vi "Recording.vi"(6 "Measurement Results In":T1 {"Actual Record Length" format="%#_6p Samples"; "Actual Record Duration" format="%#_6p Samples"; "Actual Sample Rate" format="%#_6ps"}, 7 "Recording Settings":T2={"Number of Records"=0, "Plot Names"=[], "Stream To File?"=FALSE, "TDMS Session"=refnum, "Fetch Timeout"=0.0, "Channels Per Record"=1} {"Fetch Timeout" format="%.2f"}, 8 "error in":errorcluster, 9 "Channel List":string, 10 "FGEN Session In":refnum<k15>, 11 "measurement context in":refnum<class "Measure Call Context.lvclass">) -> (0 "error out":errorcluster, 3 "measurement context out":refnum<class "Measure Call Context.lvclass">, 4 "Measurement Results Out":T1 {"Actual Record Length" format="%#_6p Samples"; "Actual Record Duration" format="%#_6ps"; "Actual Sample Rate" format="%#_6pHz"})   [LabVIEW 2025, in "Ni-Scope-Multirecords.lvclass"]
uses:
  Ni-Scope-Multirecords.lvclass
  Recording Settings.ctl
  <vilib>/Plug-In SDKs/Measurements/Measure Call Context/Measure Call Context.lvclass
  Measurement Results.ctl
  Wfm Data.ctl
  <extravilib>/ChannelInstances/Stream-t'Ni-Scope-Multirecords.lvclass-Wfm Data.ctl'/Read.vi
  <extravilib>/ChannelInstances/Stream-t'Ni-Scope-Multirecords.lvclass-Wfm Data.ctl'/Write With Abort.vi
  <extravilib>/ChannelInstances/Stream-t'Ni-Scope-Multirecords.lvclass-Wfm Data.ctl'/Read With Abort.vi
  <extravilib>/ChannelInstances/Stream-t'Ni-Scope-Multirecords.lvclass-Wfm Data.ctl'/Endpoint.vi
  <extravilib>/ChannelInstances/Stream-t'Ni-Scope-Multirecords.lvclass-Wfm Data.ctl'/EndpointRead.vi
  <extravilib>/ChannelInstances/Stream-t'Ni-Scope-Multirecords.lvclass-Wfm Data.ctl'/Instantiate.vi
  <extravilib>/ChannelInstances/Stream-t'Ni-Scope-Multirecords.lvclass-Wfm Data.ctl'/)Channel.vi
  <resource>/ChannelSupport/_ChannelSupport/WaitIfNeeded.vi
  <instrlib>/niScope/Acquire/Fetch/niScope Multi Fetch Cluster.vi
  Ni-Scope-Multirecords.lvclass/Ni-Scope-Multirecords.ctl
  <extravilib>/ChannelInstances/Stream-t'Ni-Scope-Multirecords.lvclass-Wfm Data.ctl'.lvlib
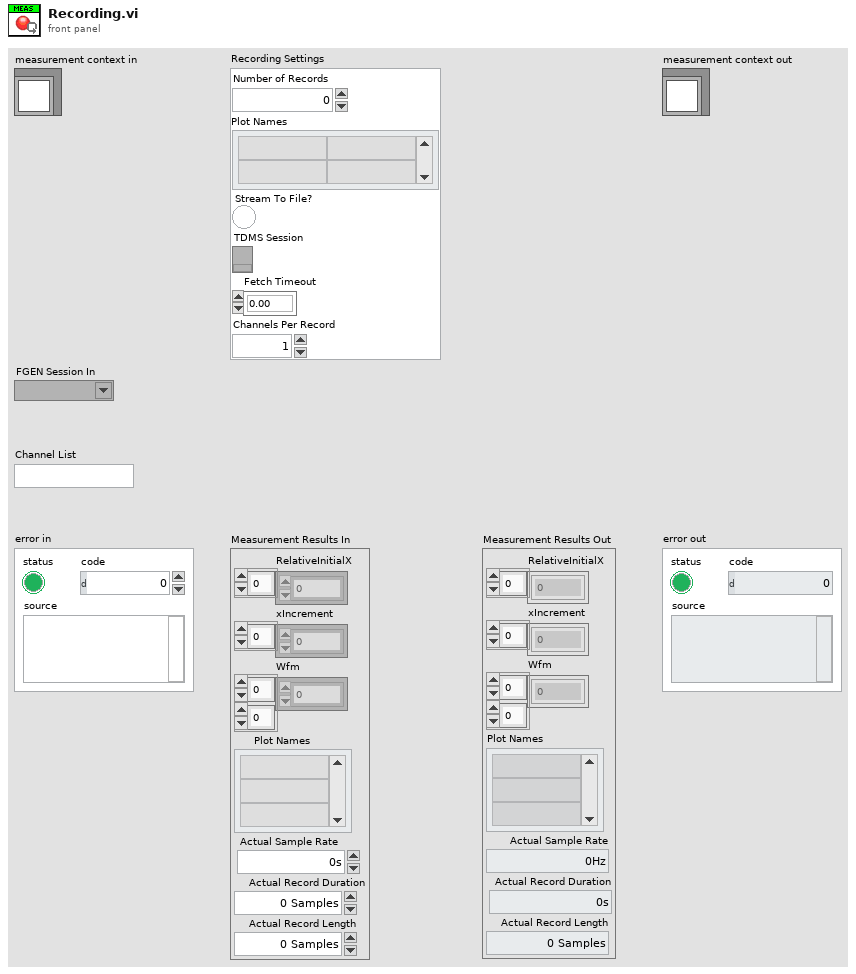
[diagram p1: front panel]
types:
  T1 = typedef "Ni-Scope-Multirecords.lvclass/Measurement Results.ctl" = cluster{"RelativeInitialX":dbl[], "xIncrement":dbl[], "Wfm":dbl[][], "Plot Names":string[], "Actual Sample Rate":dbl, "Actual Record Duration":dbl, "Actual Record Length":dbl}
  T2 = typedef "Ni-Scope-Multirecords.lvclass/Recording Settings.ctl" = cluster{"Number of Records":i32, "Plot Names":string[][], "Stream To File?":bool, "TDMS Session":refnum<k34>, "Fetch Timeout":dbl, "Channels Per Record":i32}
  T3 = typedef "Ni-Scope-Multirecords.lvclass/Wfm Data.ctl" = cluster{"waveform":cluster{"relativeInitialX":dbl, "xIncrement":dbl, "wfm":dbl[]}[]}
  T4 = cluster{"relativeInitialX":dbl, "xIncrement":dbl, "wfm":dbl[]}[]
  T5 = typedef "Stream-t'Ni-Scope-Multirecords.lvclass-Wfm Data.ctl'.lvlib/)Channel.ctl" = refnum<queue>
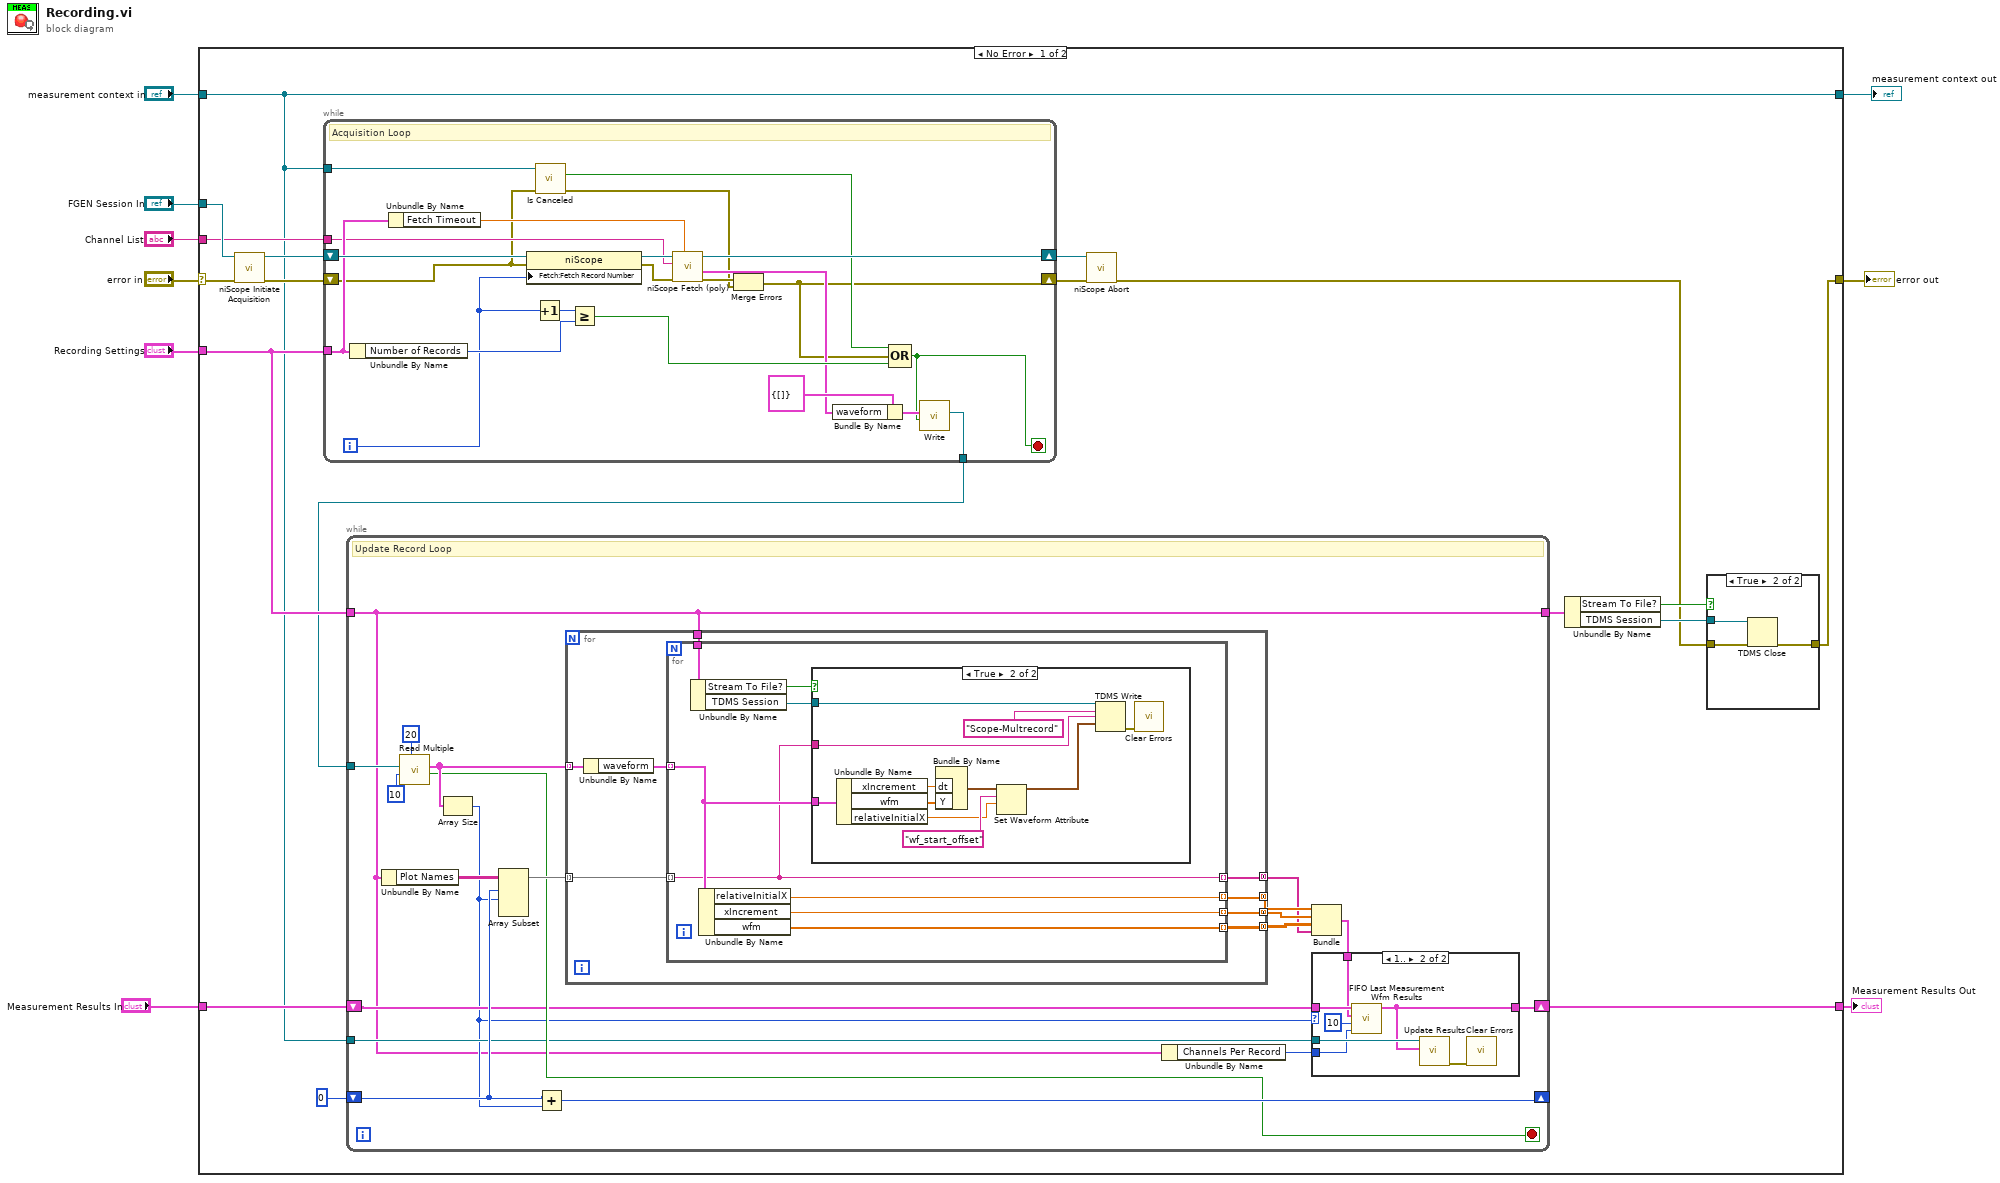
[diagram p0: block diagram]
diagram:
  n1 = case shown="No Error" "error in" {
    selector: "error in" -> [w27 w111]
    tunnel: [w10 w111] -> w8
    tunnel: "Recording Settings" -> [w23 _]
    tunnel: "measurement context in" -> [w17 w110]
    tunnel: "FGEN Session In" -> [w25 _]
    tunnel: [w17 w110] -> w4
    tunnel: "Channel List" -> [w19 _]
    tunnel: "Measurement Results In" -> [w18 w109]
    tunnel: [w16 w109] -> w1
    frame No Error {
      n2 = call <instrlib>:"niScope Initiate Acquisition.vi"("instrument handle"=w25, "error in"=w27) -> ("instrument handle out"=w26:refnum<k15>, "error out"=w24:errorcluster)  [unwired: 12 in]
      n3 = while {
        tunnel: w23 -> [w100]
        shift-right: [w106] -> w15
        shift-left: w26 -> [w108]
        shift-right: [w88] -> w20
        shift-left: w24 -> [w89]
        tunnel: w17 -> [w97]
        tunnel: [w93] -> w22
        tunnel: w19 -> [w91]
        i -> [w103]
        stop <- w92 stop-if-true
        # "Acquisition Loop"
        n4 = Unbundle By Name(w100) -> ("Number of Records"=w105:i32)
        n5 = Unbundle By Name(w100) -> ("Fetch Timeout"=w99:dbl)
        n6 = property class="niScope"(reference=w108, error in=w89, "Fetch:Fetch Record Number"=w103) -> (reference out=w107:refnum<k15>, error out=w101:errorcluster)
        n7 = Increment(x=w103) -> (x+1=w104:i32)
        n8 = call <vilib>:"Is Canceled.vi"("error in"=w89, "measure call context in"=w97) -> ("error out"=w87:errorcluster, "is canceled?"=w90:bool)  [unwired: 7 in, 1 out]
        n9 = Greater Or Equal?(x=w104, y=w105) -> (x >= y?=w102:bool)
        n10 = call-poly <instrlib>:"niScope Fetch (poly).vi"("timeout"=w99, "error in"=w101, "channels"=w91, "instrument handle"=w107) -> ("error out"=w98:errorcluster, "waveform"=w95:T4, "instrument handle out"=w106:refnum<k15>)  [unwired: 4 in, 1 out]
        n11 = Merge Errors(w98, w87) -> (w88:errorcluster)
        n12 = Bundle By Name(cluster=T3 {"waveform"=[]}, "waveform"=w95) -> (w94:T3)
        n13 = Compound Arithmetic op=OR(w90, w88, w102) -> (w92:bool)
        n14 = call <extravilib>:"Write.vi"("last element? (F)"=w92, "element"=w94) -> ("channel"=w93:T5)  [unwired: 7 in, 2 out]
      }
      n15 = while {
        tunnel: w23 -> [w32]
        tunnel: w22 -> [w50]
        shift-right: [w46] -> _
        shift-left: 0 -> [w47]
        shift-right: [w35] -> w16
        shift-left: w18 -> [w42]
        tunnel: w17 -> [w36]
        tunnel: [w32] -> w14
        stop <- w45 stop-if-true
        # "Update Record Loop"
        n16 = Unbundle By Name(w32) -> ("Plot Names"=w51:string[][])
        n17 = call <extravilib>:"Read Multiple.vi"("timeout in ms (-1)"=20, "number to read (-1, available)"=10, "channel"=w50) -> ("last element?"=w45:bool, "elements"=w48:T3[])  [unwired: 5 in, 2 out]
        n18 = Array Size(array=w48) -> (size(s)=w34:i32)
        n19 = Array Subset(array=w51, index (row)=w47, length (row)=w34) -> (w49:string[][])  [unwired: 2 in]
        n20 = Add(x=w47, y=w34) -> (x+y=w46:i32)
        n21 = for {
          tunnel: w49 -> [w66] mode=indexing
          tunnel: w48 -> [w65] mode=indexing
          tunnel: w32 -> [w64]
          tunnel: [w63] -> w41 mode=concatenating
          tunnel: [w62] -> w40 mode=concatenating
          tunnel: [w61] -> w39 mode=concatenating
          tunnel: [w60] -> w38 mode=concatenating
          n22 = Unbundle By Name(w65) -> ("waveform"=w67:T4)
          n23 = for {
            tunnel: w67 -> [w71] mode=indexing
            tunnel: [w75] -> w63 mode=indexing
            tunnel: w66 -> [w68] mode=indexing
            tunnel: w64 -> [w73]
            tunnel: [w70] -> w62 mode=indexing
            tunnel: [w69] -> w61 mode=indexing
            tunnel: [w68] -> w60 mode=indexing
            n24 = Unbundle By Name(w73) -> ("Stream To File?"=w74:bool, "TDMS Session"=w72:refnum<k34>)
            n25 = Unbundle By Name(w71) -> ("relativeInitialX"=w75:dbl, "xIncrement"=w70:dbl, "wfm"=w69:dbl[])
            n26 = case shown="True" w74 {
              tunnel: w72 -> [_ w78]
              tunnel: w71 -> [_ w80]
              tunnel: w68 -> [_ w77]
              frame False {
              }
              frame True {
                n27 = Unbundle By Name(w80) -> ("xIncrement"=w84:dbl, "wfm"=w85:dbl[], "relativeInitialX"=w81:dbl)
                n28 = Bundle By Name("dt"=w84, "Y"=w85) -> (w83:waveform(dbl))  [unwired: 1 in]
                n29 = Set Waveform Attribute(5:w81, 6:"wf_start_offset" ("name"), 7:w83) -> (3:w79:waveform(dbl))  [unwired: 1 in, 2 out]
                n30 = TDMS Write(0:w78, 5:"Scope-Multrecord" ("group name in (Untitled)"), 7:w77, 9:w79) -> (15:w76:errorcluster)  [unwired: 2 in, 3 out]
                n31 = call <vilib>:"Clear Errors.vi"("error in (no error)"=w76) -> ()  [unwired: 5 in, 2 out]
              }
            }
          }
        }
        n32 = Unbundle By Name(w32) -> ("Channels Per Record"=w33:i32)
        n33 = Bundle(w41, w40, "wfm"=w39, w38) -> (w37:cluster{dbl[], dbl[], "wfm":dbl[][], string[]})  [unwired: 1 in]
        n34 = case shown="1.." w34 {
          tunnel: w42 -> [w52 w59]
          tunnel: w37 -> [_ w58]
          tunnel: w36 -> [_ w56]
          tunnel: [w52 w55] -> w35
          tunnel: w33 -> [_ w53]
          frame Default {
          }
          frame 1.. {
            n35 = call "FIFO Last Measurement Wfm Results.vi"("Channels Per Record"=w53, "Record Upper Limit"=10 ("Upper Limit"), "New Data"=w58, "measurement results in"=w59) -> ("measurement results out"=w55:T1)  [unwired: 7 in]
            n36 = call <vilib>:"Update Results.vi"("measurement results"=w55, "measure call context in"=w56) -> ("error out"=w54:errorcluster)  [unwired: 8 in, 1 out]
            n37 = call <vilib>:"Clear Errors.vi"("error in (no error)"=w54) -> ()  [unwired: 5 in, 2 out]
          }
        }
      }
      n38 = call <instrlib>:"niScope Abort.vi"("instrument handle"=w15, "error in"=w20) -> ("error out"=w11:errorcluster)  [unwired: 12 in, 1 out]
      n39 = Unbundle By Name(w14) -> ("Stream To File?"=w13:bool, "TDMS Session"=w12:refnum<k34>)
      n40 = case shown="True" w13 {
        tunnel: w12 -> [_ w31]
        tunnel: w11 -> [w28 w30]
        tunnel: [w28 w29] -> w10
        frame False {
        }
        frame True {
          n41 = TDMS Close(8:w30, 11:w31) -> (0:w29:errorcluster)  [unwired: 1 out]
        }
      }
    }
    frame Error {
    }
  }
  "error out" <- w8
  "measurement context out" <- w4
  "Measurement Results Out" <- w1
